vi "Get Parameter Value - Boolean.vi"(7 "Default value":bool, 8 "error in (no error)":errorcluster, 9 "Parameter name":string, 10 "Config name":string, 11 "Config in":refnum<class "Config.lvclass">) -> (0 "error out":errorcluster, 2 "Value":bool, 3 "Config out":refnum<class "Config.lvclass">)   [LabVIEW 2026, in "TALOS.lvlib" / "Classes.lvlib" / "Config.lvclass"]
doc: "Get the parameter's value (double) from the specified configuration"
uses:
  Config.lvclass
  Ancestor/Ancestor/Ancestor.lvclass/Ancestor.ctl
  FGV/Error Memory/Get Error Description.vi
  Support VIs/Get PC name.vi
  Ancestor/Ancestor/Read ID.vi
  Support VIs/Get Class Name.vi
  <vilib>/Utility/error.llb/Clear Errors.vi
  FGV/Error Memory/Error Memory Core.vi
  <vilib>/AdvancedString/Delimited String to 1D String Array.vi
  <vilib>/AdvancedString/Delimited String to 1D String Array (string).vi
  Support VIs/Circus Root Path.vi
  FGV/Error Memory/Error Crt Lvl checker.vi
  FGV/Error Memory/Error Memory Core.vi/40c8088d-b597-4017-91af-faa98e00292e.vi
  FGV/Error Memory/Error Memory Core.vi/d4a3ab98-063c-4e44-b43d-fbdcfe6c2be2.vi
  Support VIs/Global Memory.vi
  <vilib>/Utility/LVClass/Get LV Class Name.vi
  Support VIs/Is in Packed Library.vi
  Support VIs/TALOS Root path.vi
  Support VIs/Read CSV worksheet.vi
  Support VIs/Global Constants.vi
  <vilib>/Utility/error.llb/General Error Handler.vi
  Ancestor/Ancestor/Ancestor.lvclass
  <vilib>/Comparison/Equal/Equal Functor/Equal Functor.lvclass
  TALOS.lvlib
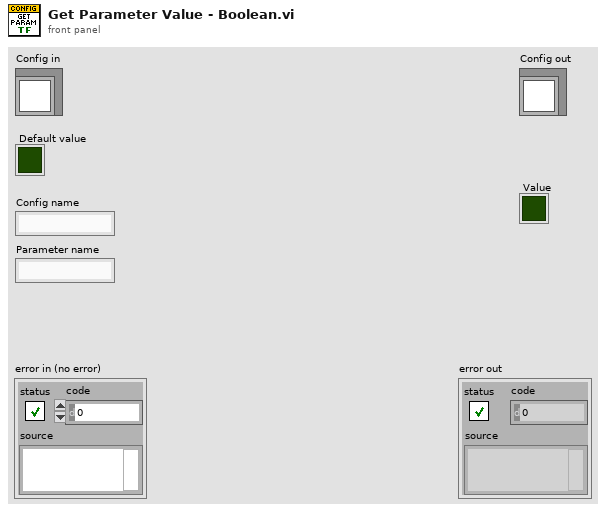
[diagram p1: front panel]
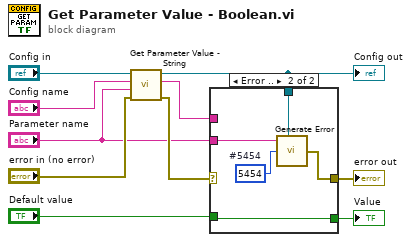
[diagram p0: block diagram]
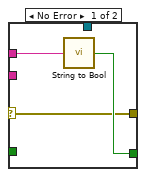
[diagram p2: hidden frame]
diagram:
  n1 = call "Get Parameter Value - String.vi"("error in (no error)"="error in (no error)", "Parameter name"="Parameter name", "Config name"="Config name", "Config in"="Config in") -> ("error out"=w7:errorcluster, "Value"=w1:string, "Config out"=w4:refnum<class "Config.lvclass">)  [unwired: 5 in]
  "Config out" <- w4
  n2 = case shown="Error .." w7 {
    selector: w7 -> [w11 _]
    tunnel: [w12 w14] -> w3
    tunnel: w4 -> [_ w17]
    tunnel: [w11 w18] -> w2
    tunnel: "Default value" -> [_ w14]
    tunnel: "Parameter name" -> [_ w15]
    tunnel: w1 -> [w13 _]
    frame No Error {
      n3 = call "String to Bool.vi"("String"=w13) -> ("Boolean"=w12:bool)
    }
    frame Error {
      w16 = 5454  # #5454
      n4 = call "Generate Error.vi"("Optional String"=w15, "Class"=w17, "Error Code"=w16) -> ("error out"=w18:errorcluster)  [unwired: 4 in]
    }
  }
  "error out" <- w2
  "Value" <- w3
